vi "WithParent_TreeHasTag.vi"() -> (0 "error out":errorcluster)   [LabVIEW 2017, in "ResultTree.Tests.lvlib" / "AddTestSuite.lvlib"]
uses:
  AddTestSuite.lvlib
  2a6c7ef5-d8ea-4de4-ba7d-c6663dbf2225.vi
  Constraint/IsEqual/Create.vi
  Constraint/IsEqual/IsEqual.lvclass
  ResultTree/ResultTree.lvclass
panel:
  in  "Tree":string(tree)
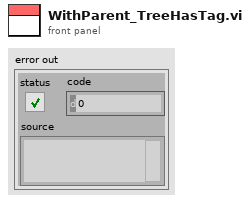
[diagram p1: front panel]
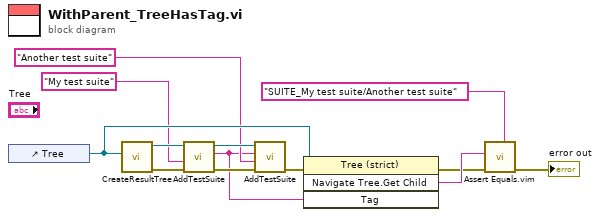
[diagram p0: block diagram]
diagram:
  n1 = control-ref of="Tree"() -> (w12:refnum<vi>)
  n2 = call "CreateResultTree.vi"("Tree Refnum"=w12) -> ("error out"=w11:errorcluster, "ResultTree out"=w10:refnum<class "ResultTree.lvclass">)  [unwired: 9 in]
  n3 = call "AddTestSuite.vi"("error in (no error)"=w11, "Name"="My test suite", "ResultTree in"=w10) -> ("error out"=w5:errorcluster, "Tag Name"=w1:string, "ResultTree out"=w6:refnum<class "ResultTree.lvclass">)  [unwired: 6 in]
  n4 = call "AddTestSuite.vi"("error in (no error)"=w5, "Name"="Another test suite", "Parent Tag (\"\")"=w1, "ResultTree in"=w6) -> ("error out"=w4:errorcluster)  [unwired: 5 in, 2 out]
  n5 = invoke class="Tree (strict)" method="Navigate Tree.Get Child"(reference=w12, error in=w4, "Tag"=w1) -> (error out=w8:errorcluster, "Navigate Tree:Get Child"=w9:string)  [unwired: 1 in, 2 out]
  n6 = call "Assert Equals.vim"("Expected"="SUITE_My test suite/Another test suite" ("Name"), "error in (no error)"=w8, "Actual"=w9) -> ("error out"=→"error out":errorcluster)  [unwired: 8 in]
